vi "AbortHardware.vi"(8 "error in (no error)":errorcluster, 11 "XPS-RLD.lvclass":refnum<class "XPS-RLD.lvclass">) -> (0 "error out":errorcluster)   [LabVIEW 2020]
uses:
  XPS-RLD.lvclass
  C:/GEECS/Developers Version/source/Device Drivers/NewportXPS/NewportXPS.lvclass
  C:/GEECS/Developers Version/source/Device Drivers/BaseDriver/BaseDriver.lvclass
  C:/GEECS/Developers Version/source/Device Drivers/NewportXPS/XPS-RLD/XPS-RLD.lvclass
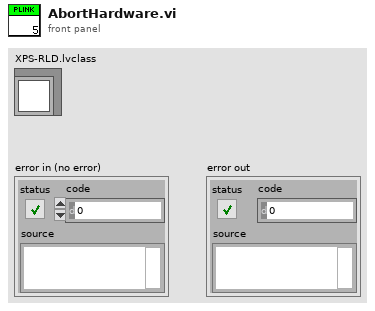
[diagram p1: front panel]
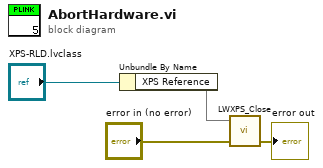
[diagram p0: block diagram]
diagram:
  n1 = Unbundle By Name("XPS-RLD.lvclass") -> ("XPS Reference"=w4)
  n2 = call "LWXPS_Close.vi"("LabVIEW error IN"="error in (no error)", "CommandInterfaceXPS.XPS"=w4) -> ("LabVIEW error OUT"=→"error out":errorcluster)  [unwired: 2 in, 1 out]
